vi "Read(Monitor).vi"(8 "error in (no error)":errorcluster, 11 "VISA resource name":refnum<visa-resource-name>) -> (0 "error out":errorcluster, 1 "Monitor2 Value":dbl, 2 "Monitor1 Value":dbl, 3 "VISA resource name out":refnum<visa-resource-name>)   [LabVIEW 2014, in "LCR Meter.lvlib"]
doc: "Query the the latest measurement data of the moniter1 and moniter2 parameters into the output buffer."
uses:
  <instrlib>/LCR Meter/Examples/LCR Meter Acquire Single_1 Folder/LCR Meter.lvlib
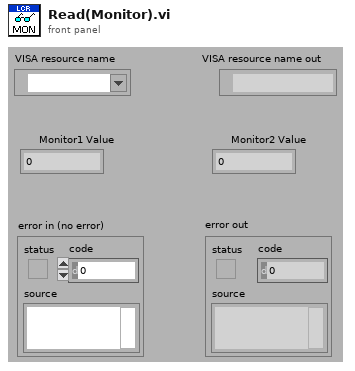
[diagram p1: front panel]
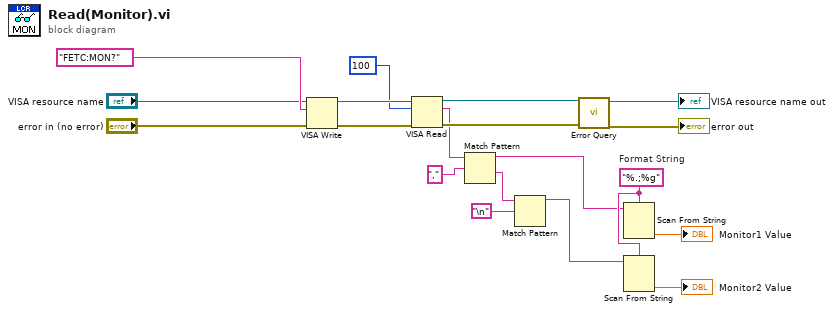
[diagram p0: block diagram]
diagram:
  w3 = "%.;%g"  # Format String
  n1 = VISA Write(VISA resource name="VISA resource name", write buffer="FETC:MON?", error in (no error)="error in (no error)") -> (VISA resource name out=w14:refnum<visa-resource-name>, error out=w13:errorcluster)  [unwired: 1 out]
  n2 = VISA Read(VISA resource name=w14, byte count=u32 100, error in (no error)=w13) -> (VISA resource name out=w12:refnum<visa-resource-name>, read buffer=w9:string, error out=w11:errorcluster)  [unwired: 1 out]
  n3 = Match Pattern(string=w9, regular expression=",") -> (before substring=w2:string, after substring=w7:string)  [unwired: 1 in, 2 out]
  n4 = Match Pattern(string=w7, regular expression="\n") -> (before substring=w1:string)  [unwired: 1 in, 3 out]
  n5 = call <instrlib>:"Error Query.vi"("error in (no error)"=w11, "VISA resource name"=w12) -> ("error out"=→"error out":errorcluster, "VISA resource name out"=→"VISA resource name out":refnum<visa-resource-name>)  [unwired: 6 in, 2 out]
  n6 = Scan From String(format string=w3, input string=w2) -> (output 1=→"Monitor1 Value":dbl)  [unwired: 3 in, 3 out]
  n7 = Scan From String(format string=w3, input string=w1) -> (output 1=→"Monitor2 Value":dbl)  [unwired: 3 in, 3 out]
